vi "TRAN-READ.vi"(8 "error in (no error)":errorcluster, 10 "Numero de transd":u64[](array[numeric]), 11 "ARRAY IN":string[](array[string])) -> (0 "error out":errorcluster, 1 "Valor Transductores":u16[](array[numeric]))   [LabVIEW 2014, in "CAP-USB.lvlib"]
doc: "Vi encargado de procesar los 2 datos por transductor enviados por \nel CAP-USB."
uses:
  CAP-USB.lvlib
  0-Nivel/Enum DI-Reader.ctl
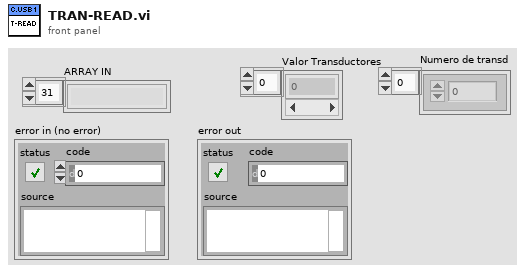
[diagram p1: front panel]
types:
  T1 = typedef "CAP-USB.lvlib/Enum DI-Reader.ctl" = enum16{"IDLE", "Detect XX", "Detect YY", "Valor", ""}
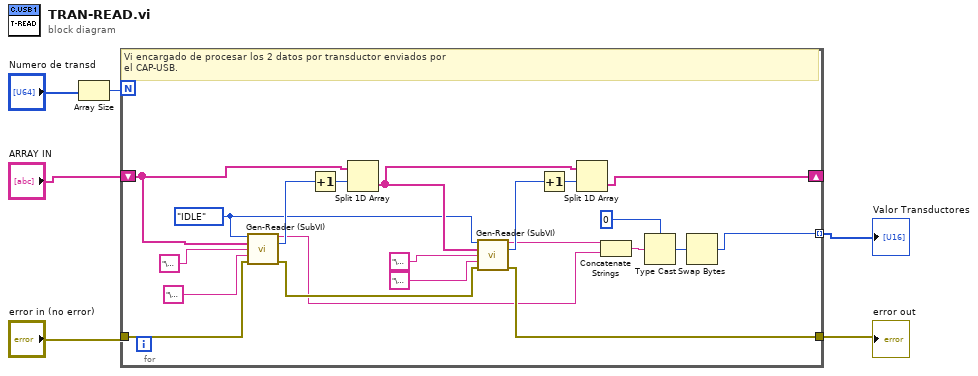
[diagram p0: block diagram]
diagram:
  n1 = Array Size(array="Numero de transd") -> (size(s)=w2:i32)
  n2 = for {
    N: w2 -> [_]
    shift-right: [w20] -> _
    shift-left: "ARRAY IN" -> [w21]
    tunnel: "error in (no error)" -> [w27]
    tunnel: [w26] -> w3
    tunnel: [w7] -> w1 mode=indexing
    w8 = Enum_DI-Reader."IDLE"
    # "Vi encargado de procesar los 2 datos por transductor enviados por \nel CAP-USB."
    n3 = call "Gen-Reader (SubVI).vi"("Enum"=w8, "ARRAY IN"=w21, "XX"="\u0003", "YY"="\u0010", "error in (no error)"=w27) -> ("read buffer"=w10:string, "Index+1"=w16:i32, "error out"=w23:errorcluster)  [unwired: 8 in]
    n4 = Increment(x=w16) -> (x+1=w15:i32)
    n5 = Split 1D Array(array=w21, index=w15) -> (second subarray=w22:string[])  [unwired: 1 out]
    n6 = call "Gen-Reader (SubVI).vi"("Enum"=w8, "ARRAY IN"=w22, "XX"="\u0003", "YY"="\u0010", "error in (no error)"=w23) -> ("read buffer"=w9:string, "Index+1"=w11:i32, "error out"=w26:errorcluster)  [unwired: 8 in]
    n7 = Increment(x=w11) -> (x+1=w12:i32)
    n8 = Split 1D Array(array=w22, index=w12) -> (second subarray=w20:string[])  [unwired: 1 out]
    n9 = Concatenate Strings(w9, w10) -> (w25:string)
    n10 = Type Cast(type=u16 0 ("default (0 U32)"), x=w25) -> (*(type *) &x=w19:u16)
    n11 = Swap Bytes(anything=w19) -> (byte swapped=w7:u16)
  }
  "error out" <- w3
  "Valor Transductores" <- w1
